vi "Reset Expected Heartbeat.vi"(8 "Error In":errorcluster, 10 "CANopen Message":refnum<class "CANopen Response Message.lvclass">, 11 "reference in":refnum<class "Network Mangement.lvclass">) -> (0 "Error Out":errorcluster, 3 "reference out":refnum<class "Network Mangement.lvclass">)   [LabVIEW 2024, in "CANopen Master.lvlib" / "Network Mangement.lvclass"]
uses:
  Network Mangement.lvclass
  Network Mangement.lvclass/Network Mangement.ctl
  CANopen Message/CANopen Message.lvclass
  <vilib>/Utility/miscctls.llb/LVMapReplaceAction.ctl
  CANopen Response/CANopen Response Message.lvclass
  D:/git/CANopen-XNET/CANopen Message/CANopen Message.lvclass
  D:/git/CANopen-XNET/CANopen Response/CANopen Response Message.lvclass
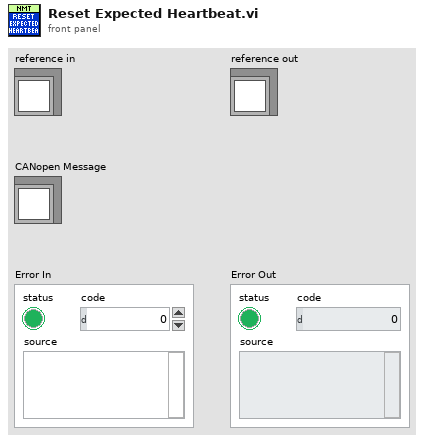
[diagram p1: front panel]
types:
  T1 = typedef "CANopen Master.lvlib/CANopen Response Message.lvclass/Server Command Specifier.ctl" = enum8{"Upload Segment Response", "Download Segment Response", "Initiate Upload Response", "Initiate Download Response", "Heartbeat", "Block Download"}
  T2 = typedef "LVMapReplaceAction.ctl" = enum32{"Modify Entry only if found", "Add or Modify Entry", "Delete Entry"}
  T3 = typedef "CANopen Master.lvlib/Network Mangement.lvclass/ObjectAttributes.ctl" = cluster{"Nodes":map{u8, u8}, "Heartbeats":map{u8, cluster{"Period":u16, "Timeout":u16, "Last Beat":timestamp}}}
  T4 = map{u8, cluster{"Period":u16, "Timeout":u16, "Last Beat":timestamp}}
  T5 = cluster{"Period":u16, "Timeout":u16, "Last Beat":timestamp}
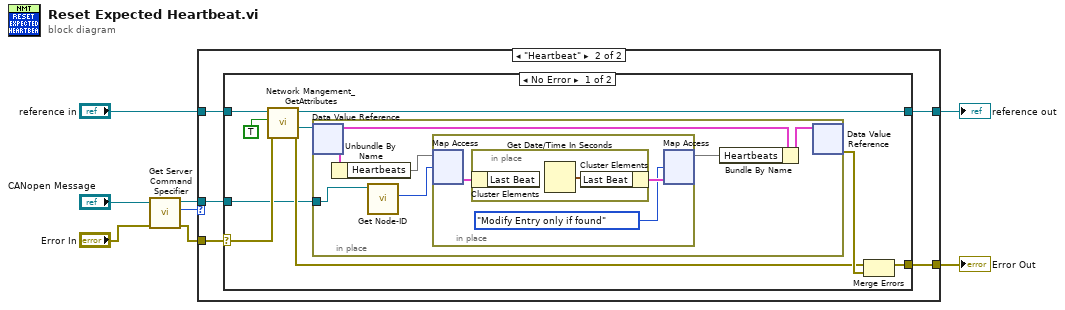
[diagram p0: block diagram]
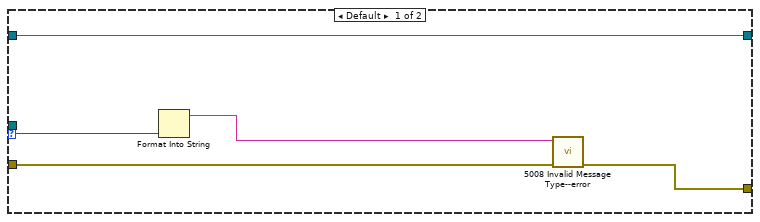
[diagram p2: hidden frame]
diagram:
  n1 = call-dynamic "Get Server Command Specifier.vi"("error in"="Error In", "CANopen Response in"="CANopen Message") -> ("error out"=w3:errorcluster, "Server Command Specifier"=w2:T1, "CANopen Response out"=w1:refnum<class "CANopen Response Message.lvclass">)  [unwired: 7 in]
  n2 = case shown="\"Heartbeat\"" w2 {
    selector: w2 -> [w11 _]
    tunnel: [w12 w18] -> w8
    tunnel: "reference in" -> [w9 w17]
    tunnel: [w9 w16] -> w6
    tunnel: w3 -> [w13 w15]
    tunnel: w1 -> [_ w14]
    frame Default {
      n3 = Format Into String(w11) -> (resulting string=w10:string)  [unwired: 3 in, 1 out]
      n4 = call "5008 Invalid Message Type--error.vi"("error in"=w13, "Argument"=w10) -> ("error out"=w12:errorcluster)  [unwired: 9 in]
    }
    frame "Heartbeat" {
      n5 = case shown="No Error" w15 {
        selector: w15 -> [w26 w39]
        tunnel: [w23 w39] -> w18
        tunnel: [w24 w38] -> w16
        tunnel: w17 -> [w27 w38]
        tunnel: w14 -> [w19 _]
        frame No Error {
          n6 = call "Network Mangement_GetAttributes.vi"("Error In"=w26, "OnlyGetDvrReference(False)"=TRUE, "reference in"=w27) -> ("Error Out"=w21:errorcluster, "DataRef"=w22:refnum<data-value>, "reference out"=w24:refnum<class "Network Mangement.lvclass">)  [unwired: 5 in, 1 out]
          n7 = in-place {
            in-place-border: w19 -> [w31]
            n8 = in-place-dvr #1(w22) -> (w32:T3)  [unwired: 1 out]
            n9 = Unbundle By Name(w32) -> ("Heartbeats"=w30:T4)
            n10 = call "Get Node-ID.vi"("CANopen Message in"=w31) -> ("Node-ID"=w29:u8)  [unwired: 9 in, 1 out]
            n11 = in-place {
              n12 = in-place-map #2(w30, w29) -> (w36:T5)  [unwired: 1 in, 1 out]
              n13 = in-place {
                n14 = in-place-cluster #3(w36) -> ()  [unwired: 1 out]
                n15 = Get Date/Time In Seconds() -> (seconds since 1Jan1904=w37:timestamp)
                n16 = in-place-cluster #3("Last Beat"=w37) -> (w35:T5)
              }
              n17 = in-place-map #2(w35, LVMapReplaceAction."Modify Entry only if found" ("action")) -> (w28:T4)  [unwired: 2 out]
            }
            n18 = Bundle By Name(cluster=w32, "Heartbeats"=w28) -> (w33:T3)
            n19 = in-place-dvr #1(w33) -> (w25:errorcluster)  [unwired: 1 out]
          }
          n20 = Merge Errors(w21, w25) -> (w23:errorcluster)
        }
        frame Error {
        }
      }
    }
  }
  "Error Out" <- w8
  "reference out" <- w6
